vi "Version_4.9_8_on-chip_valves_for25ulSyringe_withModfied_Plunging.vi"() -> ()   [LabVIEW 2020] (continued)
                              tunnel: w4033 -> [w4039]
                              tunnel: w4032 -> [w4038]
                              stop <- w4036 stop-if-true
                              n3656 = Wait (ms)(milliseconds to wait=u32 100) -> ()  [unwired: 1 out]
                              n3657 = stacked-sequence {
                                tunnel: w4041 -> [w4047 _]
                                tunnel: w4040 -> [w4046 w4069]
                                tunnel: w4039 -> [w4045 _]
                                tunnel: w4038 -> [w4044 _]
                                tunnel: [_ w4067] -> w4036
                                frame #0 {
                                n3658 = call "AbsolutePlungerPosition (SubVI).vi"("VISA Refnum in"=w4046) -> ("Plunger Position"=w4043:i32)  [unwired: 10 in]
                                n3659 = case shown="\"Standard Pumping\", Default" w4045 {
                                tunnel: w4047 -> [w4052 w4061]
                                tunnel: w4043 -> [w4053 w4060]
                                tunnel: [w4051 w4058] -> w4042
                                tunnel: w4044 -> [w4050 w4059]
                                frame "Standard Pumping", Default {
                                n3660 = Subtract(x=w4052, y=w4053) -> (x-y=w4049:dbl)
                                n3661 = Absolute Value(x=w4049) -> (abs(x)=w4048:dbl)
                                n3662 = Multiply(x=w4048, y=w4050) -> (x*y=w4055:dbl)
                                n3663 = Divide(x=w4055, y=3000.0) -> (x/y=w4051:dbl)
                                }
                                frame "High Resolution Pumping" {
                                n3664 = Subtract(x=w4061, y=w4060) -> (x-y=w4057:dbl)
                                n3665 = Absolute Value(x=w4057) -> (abs(x)=w4056:dbl)
                                n3666 = Multiply(x=w4056, y=w4059) -> (x*y=w4063:dbl)
                                n3667 = Divide(x=w4063, y=24000.0) -> (x/y=w4058:dbl)
                                }
                                }
                                n3668 = local write "Volume being Injected \nin this process"(w4042) -> ()
                                }
                                frame #1 {
                                n3669 = call "LSPOneStatus (SubVI).vi"("VISA Refnum in"=w4069) -> ("read buffer"=w4071:string)  [unwired: 10 in]
                                n3670 = call <vilib>:"Trim Whitespace.vi"("string"=w4071) -> ("trimmed string"=w4070:string)  [unwired: 1 in]
                                n3671 = Equal?(x=w4070, y="/0`\u0003") -> (x = y?=w4068:bool)
                                n3672 = local read "Stopper that ends \nthe main loops"() -> (w4065:bool)
                                n3673 = local read "Divert Sample \nonto Grid"() -> (w4066:bool)
                                n3674 = Or(x=w4066, y=w4065) -> (x .or. y?=w4064:bool)
                                n3675 = Or(x=w4068, y=w4064) -> (x .or. y?=w4067:bool)
                                }
                              }
                            }
                            n3676 = local read "Stopper that ends \nthe main loops"() -> (w4031:bool)
                            n3677 = case shown="True" w4031 {
                              frame False {
                              }
                              frame True {
                                n3678 = local read "VISA Refnum in\nfor Pump"() -> (w4073:refnum<visa-resource-name>)
                                n3679 = call "HardStopCurrentProcess (SubVI).vi"("VISA Refnum in"=w4073) -> ()  [unwired: 11 in]
                              }
                            }
                          }
                          frame #30 {
                            n3680 = local read "Volume being Injected \nin this process"() -> (w4076:dbl)
                            n3681 = local read "VISA Refnum in\nfor Pump"() -> (w4078:refnum<visa-resource-name>)
                            n3682 = call "AbsolutePlungerPosition (SubVI).vi"("VISA Refnum in"=w4078) -> ("Plunger Position"=w4077:i32)  [unwired: 10 in]
                            n3683 = local write "Pause Data Collection"(TRUE) -> ()
                            n3684 = local write "True Volume being \ninjected in this\nprocess"(w4076) -> ()
                            n3685 = local write "Position\nNow"(w4077) -> ()
                            n3686 = Wait (ms)(milliseconds to wait=u32 500) -> ()  [unwired: 1 out]
                          }
                          frame #31 {
                            # "Sample Deposition onto EM-Grid"
                            n3687 = local read "Divert Sample \nonto Grid"() -> (w4079:bool)
                            n3688 = case shown="True" w4079 {
                              frame False {
                              }
                              frame True {
                                n3689 = stacked-sequence {
                                frame #0 {
                                # "Discard the initial volume of fluid that is present in the channel prior to detection"
                                n3690 = local read "Buffer-C2 Pumping\nResolution"() -> (w4090:T2)
                                n3691 = local read "Initial Plunger Position"() -> (w4089:dbl)
                                n3692 = local read "VISA Refnum in\nfor Pump"() -> (w4091:refnum<visa-resource-name>)
                                n3693 = local read "Position\nNow"() -> (w4087:dbl)
                                n3694 = local read "Volume of Syringe"() -> (w4088:dbl)
                                n3695 = local write "Pause Data Collection"(FALSE) -> ()
                                n3696 = while {
                                tunnel: w4091 -> [w4101]
                                tunnel: w4090 -> [w4100]
                                tunnel: w4089 -> [w4096]
                                tunnel: w4088 -> [w4099]
                                tunnel: w4087 -> [w4095]
                                stop <- w4097 stop-if-true
                                n3697 = stacked-sequence {
                                tunnel: w4101 -> [w4107 w4129 w4159]
                                tunnel: w4100 -> [w4106 w4128 _]
                                tunnel: w4096 -> [w4104 _ _]
                                tunnel: w4099 -> [w4103 w4126 _]
                                tunnel: [_ _ w4152] -> w4097
                                tunnel: w4095 -> [_ w4124 _]
                                frame #0 {
                                # "From here on 'True Volume being injected \nin this process' represents the true total \nvolume in this process"
                                n3698 = call "AbsolutePlungerPosition (SubVI).vi"("VISA Refnum in"=w4107) -> ("Plunger Position"=w4105:i32)  [unwired: 10 in]
                                n3699 = case shown="..\"Standard Pumping\"" w4106 {
                                tunnel: w4105 -> [w4115 w4123]
                                tunnel: w4104 -> [w4114 w4122]
                                tunnel: w4103 -> [w4111 w4119]
                                tunnel: [w4108 w4116] -> w4102
                                frame .."Standard Pumping" {
                                n3700 = Subtract(x=w4115, y=w4114) -> (x-y=w4113:dbl)
                                n3701 = Absolute Value(x=w4113) -> (abs(x)=w4112:dbl)
                                n3702 = Multiply(x=w4112, y=w4111) -> (x*y=w4110:dbl)
                                n3703 = Divide(x=w4110, y=3000.0) -> (x/y=w4108:dbl)
                                }
                                frame "High Resolution Pumping".. {
                                n3704 = Subtract(x=w4123, y=w4122) -> (x-y=w4121:dbl)
                                n3705 = Absolute Value(x=w4121) -> (abs(x)=w4120:dbl)
                                n3706 = Multiply(x=w4120, y=w4119) -> (x*y=w4118:dbl)
                                n3707 = Divide(x=w4118, y=24000.0) -> (x/y=w4116:dbl)
                                }
                                }
                                n3708 = local write "True Volume being \ninjected in this\nprocess"(w4102) -> ()
                                }
                                frame #1 {
                                # "From here on 'Volume being injected \nin this process' represents the volume \nin this sub process"
                                n3709 = call "AbsolutePlungerPosition (SubVI).vi"("VISA Refnum in"=w4129) -> ("Plunger Position"=w4127:i32)  [unwired: 10 in]
                                n3710 = case shown="..\"Standard Pumping\"" w4128 {
                                tunnel: w4127 -> [w4137 w4145]
                                tunnel: w4124 -> [w4136 w4144]
                                tunnel: w4126 -> [w4133 w4141]
                                tunnel: [w4130 w4138] -> w4125
                                frame .."Standard Pumping" {
                                n3711 = Subtract(x=w4137, y=w4136) -> (x-y=w4135:dbl)
                                n3712 = Absolute Value(x=w4135) -> (abs(x)=w4134:dbl)
                                n3713 = Multiply(x=w4134, y=w4133) -> (x*y=w4132:dbl)
                                n3714 = Divide(x=w4132, y=3000.0) -> (x/y=w4130:dbl)
                                }
                                frame "High Resolution Pumping".. {
                                n3715 = Subtract(x=w4145, y=w4144) -> (x-y=w4143:dbl)
                                n3716 = Absolute Value(x=w4143) -> (abs(x)=w4142:dbl)
                                n3717 = Multiply(x=w4142, y=w4141) -> (x*y=w4140:dbl)
                                n3718 = Divide(x=w4140, y=24000.0) -> (x/y=w4138:dbl)
                                }
                                }
                                n3719 = local write "Volume being Injected \nin this process"(w4125) -> ()
                                }
                                frame #2 {
                                n3720 = local read "Discard Volume"() -> (w4146:dbl)
                                n3721 = local read "Discard fluid \nprior to 1st \ndeposition"() -> (w4151:bool)
                                n3722 = local read "Volume being Injected \nin this process"() -> (w4150:dbl)
                                n3723 = Greater Or Equal?(x=w4150, y=w4146) -> (x >= y?=w4148:bool)
                                n3724 = call "AbsolutePlungerPositionStatus (SubVI).vi"("VISA Refnum in"=w4159) -> ("read buffer"=w4158:string)  [unwired: 10 in]
                                n3725 = local read "Stop for End of \nExperiment \nand Data Writing"() -> (w4155:bool)
                                n3726 = call <vilib>:"Trim Whitespace.vi"("string"=w4158) -> ("trimmed string"=w4157:string)  [unwired: 1 in]
                                n3727 = Not(x=w4151) -> (.not. x?=w4149:bool)
                                n3728 = Equal?(x=w4157, y="/0`\u0003") -> (x = y?=w4154:bool)
                                n3729 = Or(x=w4149, y=w4148) -> (x .or. y?=w4147:bool)
                                n3730 = Or(x=w4147, y=w4155) -> (x .or. y?=w4153:bool)
                                n3731 = Or(x=w4154, y=w4153) -> (x .or. y?=w4152:bool)
                                }
                                }
                                n3732 = Wait (ms)(milliseconds to wait=u32 100) -> ()  [unwired: 1 out]
                                }
                                n3733 = local write "Valve V4 Open"(TRUE ("Valve V4 Open")) -> ()
                                n3734 = local write "Valve V3 Open"(FALSE ("Valve V3 Open")) -> ()
                                n3735 = local write "Valve V2 Open"(FALSE ("Valve V2 Open")) -> ()
                                n3736 = local write "Valve V1 Open"(FALSE ("Valve V1 Open")) -> ()
                                n3737 = local write "Valve V5 Open"(TRUE ("Valve V5 Open")) -> ()
                                n3738 = local write "Valve V6 Open"(TRUE ("Valve V6 Open")) -> ()
                                n3739 = local write "Valve V7 Open"(FALSE ("Valve V7 Open")) -> ()
                                n3740 = local write "Volume being Injected \nin this process"(0.0) -> ()
                                }
                                frame #1 {
                                # "Keeps the on-chip valve V1, V2 and V3 closed,\nHalts also deposition onto the grid\nand waits for the 1st redeposit command. Once the command is issued\nit starts pumpoing and moves onto the next frame"
                                n3741 = stacked-sequence {
                                frame #0 {
                                n3742 = local write "Valve V5 Open"(FALSE ("Valve V5 Open")) -> ()
                                n3743 = local write "Valve V1 Open"(FALSE ("Valve V1 Open")) -> ()
                                n3744 = local read "VISA Refnum in\nfor Pump"() -> (w4169:refnum<visa-resource-name>)
                                n3745 = local write "Valve V2 Open"(FALSE ("Valve V2 Open")) -> ()
                                n3746 = local write "Valve V6 Open"(FALSE ("Valve V6 Open")) -> ()
                                n3747 = local write "Re-deposit Sample\nonto Grid"(FALSE ("Redeposit Sample\nonto Grid")) -> ()
                                n3748 = local write "Pause Data Collection"(TRUE ("Pause Data Collection")) -> ()
                                n3749 = call "HardStopCurrentProcess (SubVI).vi"("VISA Refnum in"=w4169) -> ()  [unwired: 11 in]
                                n3750 = local write "Valve V7 Open"(FALSE ("Valve V7 Open")) -> ()
                                n3751 = local write "Valve V3 Open"(FALSE ("Valve V3 Open")) -> ()
                                n3752 = local write "Valve V4 Open"(FALSE ("Valve V4 Open")) -> ()
                                }
                                frame #1 {
                                n3753 = while {
                                stop <- w4172 stop-if-true
                                n3754 = local read "Stop for End of \nExperiment \nand Data Writing"() -> (w4173:bool)
                                n3755 = local read "Re-deposit Sample\nonto Grid"() -> (w4174:bool)
                                n3756 = Or(x=w4174, y=w4173) -> (x .or. y?=w4172:bool)
                                }
                                n3757 = local write "Discard fluid \nprior to 1st \ndeposition"(FALSE ("Discard fluid \nprior to 1st \ndeposition")) -> ()
                                n3758 = One Button Dialog(message="Do you want to deposit sample on another grid? If yes, turn on 'Re-deposit Sample onto Grid'. Else turn on STOP ") -> ()  [unwired: 1 in, 1 out]
                                }
                                frame #2 {
                                n3759 = local write "Valve V6 Open"(TRUE ("Valve V3 Open")) -> ()
                                n3760 = local write "Valve V4 Open"(TRUE ("Valve V1 Open")) -> ()
                                n3761 = local write "Valve V5 Open"(TRUE ("Valve V2 Open")) -> ()
                                n3762 = local write "Valve V7 Open"(FALSE ("Valve V7 Open")) -> ()
                                }
                                frame #3 {
                                n3763 = local read "Re-deposit Sample\nonto Grid"() -> (w4179:bool)
                                n3764 = case shown="True" w4179 {
                                frame False {
                                n3765 = local write "Suction On/Off"(FALSE ("Suction On/Off")) -> ()
                                }
                                frame True {
                                n3766 = stacked-sequence {
                                frame #0 {
                                n3767 = local read "VISA Refnum in\nfor Pump"() -> (w4182:refnum<visa-resource-name>)
                                n3768 = call "AbsolutePlungerPosition (SubVI).vi"("VISA Refnum in"=w4182) -> ("Plunger Position"=w4181:i32)  [unwired: 10 in]
                                n3769 = local write "Position\nNow"(w4181) -> ()
                                }
                                frame #1 {
                                n3770 = local read "Buffer-C2 Pumping\nResolution"() -> (w4184:T2)
                                n3771 = case shown="\"Standard Pumping\", Default" w4184 {
                                tunnel: [w4185 w4196] -> w4183
                                frame "Standard Pumping", Default {
                                n3772 = local read "Buffer-C2 Volume \nto be Pumped"() -> (w4188:dbl)
                                n3773 = local read "Volume of Syringe"() -> (w4191:dbl)
                                n3774 = local read "Initial Plunger Position"() -> (w4195:dbl)
                                n3775 = local read "Position\nNow"() -> (w4194:dbl)
                                n3776 = Subtract(x=w4195, y=w4194) -> (x-y=w4193:dbl)
                                n3777 = Absolute Value(x=w4193) -> (abs(x)=w4192:dbl)
                                n3778 = Multiply(x=w4192, y=w4191) -> (x*y=w4190:dbl)
                                n3779 = Divide(x=w4190, y=3000.0) -> (x/y=w4187:dbl)
                                n3780 = Subtract(x=w4187, y=w4188) -> (x-y=w4186:dbl)
                                n3781 = Absolute Value(x=w4186) -> (abs(x)=w4185:dbl)
                                }
                                frame "High Resolution Pumping" {
                                n3782 = local read "Buffer-C2 Volume \nto be Pumped"() -> (w4199:dbl)
                                n3783 = local read "Volume of Syringe"() -> (w4202:dbl)
                                n3784 = local read "Initial Plunger Position"() -> (w4206:dbl)
                                n3785 = local read "Position\nNow"() -> (w4205:dbl)
                                n3786 = Subtract(x=w4206, y=w4205) -> (x-y=w4204:dbl)
                                n3787 = Absolute Value(x=w4204) -> (abs(x)=w4203:dbl)
                                n3788 = Multiply(x=w4203, y=w4202) -> (x*y=w4201:dbl)
                                n3789 = Divide(x=w4201, y=24000.0) -> (x/y=w4198:dbl)
                                n3790 = Subtract(x=w4198, y=w4199) -> (x-y=w4197:dbl)
                                n3791 = Absolute Value(x=w4197) -> (abs(x)=w4196:dbl)
                                }
                                }
                                n3792 = local write "Buffer-C Volume\nleft to be Pumped"(w4183) -> ()
                                }
                                frame #2 {
                                n3793 = local read "Buffer-C2 Dispense\nFlow Rate (ul/min)"() -> (w4210:dbl)
                                n3794 = local read "Buffer-C2 Pumping\nResolution"() -> (w4209:T2)
                                n3795 = local read "VISA Refnum in\nfor Pump"() -> (w4212:refnum<visa-resource-name>)
                                n3796 = local read "Volume of Syringe"() -> (w4211:dbl)
                                n3797 = call "GoToAbsolutePosition(SubVI).vi"("Absolute Volume Position in Syringe (in ul)"=0.0, "Volume of Syringe"=w4211, "Resolution of Pumping"=w4209, "Flow Rate (ul/min)"=w4210, "VISA Refnum in"=w4212) -> ()  [unwired: 6 in, 1 out]
                                n3798 = local write "Suction On/Off"(FALSE ("Suction On/Off")) -> ()
                                }
                                }
                                }
                                }
                                }
                                frame #4 {
                                n3799 = local read "Stop for End of \nExperiment \nand Data Writing"() -> (w4213:bool)
                                n3800 = case shown="True" w4213 {
                                frame False {
                                }
                                frame True {
                                n3801 = local read "VISA Refnum in\nfor Pump"() -> (w4214:refnum<visa-resource-name>)
                                n3802 = call "HardStopCurrentProcess (SubVI).vi"("VISA Refnum in"=w4214) -> ()  [unwired: 11 in]
                                }
                                }
                                }
                                }
                                }
                                frame #2 {
                                # "Keeps the on-chip valve V1, V2 Open and V3 closed"
                                n3803 = while {
                                stop <- w4218 stop-if-true
                                n3804 = local read "Suction On/Off"() -> (w4219:bool)
                                n3805 = case shown="True" w4219 {
                                frame False {
                                n3806 = local read "Buffer-C2 Pumping\nResolution"() -> (w4225:T2)
                                n3807 = local read "Initial Plunger Position"() -> (w4224:dbl)
                                n3808 = local read "VISA Refnum in\nfor Pump"() -> (w4226:refnum<visa-resource-name>)
                                n3809 = local read "Position\nNow"() -> (w4222:dbl)
                                n3810 = local read "Volume of Syringe"() -> (w4223:dbl)
                                n3811 = local write "Volume being Injected \nin this process"(0.0) -> ()
                                n3812 = local write "Pause Data Collection"(FALSE) -> ()
                                n3813 = while {
                                tunnel: w4226 -> [w4233]
                                tunnel: w4225 -> [w4232]
                                tunnel: w4224 -> [w4228]
                                tunnel: w4223 -> [w4231]
                                tunnel: w4222 -> [w4227]
                                stop <- w4229 stop-if-true
                                n3814 = stacked-sequence {
                                tunnel: w4233 -> [w4239 w4261 w4286]
                                tunnel: w4232 -> [w4238 w4260 _]
                                tunnel: w4228 -> [w4236 _ _]
                                tunnel: w4231 -> [w4235 w4258 _]
                                tunnel: [_ _ w4278] -> w4229
                                tunnel: w4227 -> [_ w4256 _]
                                frame #0 {
                                # "From here on 'True Volume being injected \nin this process' represents the true total \nvolume in this process"
                                n3815 = call "AbsolutePlungerPosition (SubVI).vi"("VISA Refnum in"=w4239) -> ("Plunger Position"=w4237:i32)  [unwired: 10 in]
                                n3816 = case shown="..\"Standard Pumping\"" w4238 {
                                tunnel: w4237 -> [w4247 w4255]
                                tunnel: w4236 -> [w4246 w4254]
                                tunnel: w4235 -> [w4243 w4251]
                                tunnel: [w4240 w4248] -> w4234
                                frame .."Standard Pumping" {
                                n3817 = Subtract(x=w4247, y=w4246) -> (x-y=w4245:dbl)
                                n3818 = Absolute Value(x=w4245) -> (abs(x)=w4244:dbl)
                                n3819 = Multiply(x=w4244, y=w4243) -> (x*y=w4242:dbl)
                                n3820 = Divide(x=w4242, y=3000.0) -> (x/y=w4240:dbl)
                                }
                                frame "High Resolution Pumping".. {
                                n3821 = Subtract(x=w4255, y=w4254) -> (x-y=w4253:dbl)
                                n3822 = Absolute Value(x=w4253) -> (abs(x)=w4252:dbl)
                                n3823 = Multiply(x=w4252, y=w4251) -> (x*y=w4250:dbl)
                                n3824 = Divide(x=w4250, y=24000.0) -> (x/y=w4248:dbl)
                                }
                                }
                                n3825 = local write "True Volume being \ninjected in this\nprocess"(w4234) -> ()
                                }
                                frame #1 {
                                # "From here on 'Volume being injected \nin this process' represents the volume \nin this sub process"
                                n3826 = call "AbsolutePlungerPosition (SubVI).vi"("VISA Refnum in"=w4261) -> ("Plunger Position"=w4259:i32)  [unwired: 10 in]
                                n3827 = case shown="..\"Standard Pumping\"" w4260 {
                                tunnel: w4259 -> [w4269 w4277]
                                tunnel: w4256 -> [w4268 w4276]
                                tunnel: w4258 -> [w4265 w4273]
                                tunnel: [w4262 w4270] -> w4257
                                frame .."Standard Pumping" {
                                n3828 = Subtract(x=w4269, y=w4268) -> (x-y=w4267:dbl)
                                n3829 = Absolute Value(x=w4267) -> (abs(x)=w4266:dbl)
                                n3830 = Multiply(x=w4266, y=w4265) -> (x*y=w4264:dbl)
                                n3831 = Divide(x=w4264, y=3000.0) -> (x/y=w4262:dbl)
                                }
                                frame "High Resolution Pumping".. {
                                n3832 = Subtract(x=w4277, y=w4276) -> (x-y=w4275:dbl)
                                n3833 = Absolute Value(x=w4275) -> (abs(x)=w4274:dbl)
                                n3834 = Multiply(x=w4274, y=w4273) -> (x*y=w4272:dbl)
                                n3835 = Divide(x=w4272, y=24000.0) -> (x/y=w4270:dbl)
                                }
                                }
                                n3836 = local write "Volume being Injected \nin this process"(w4257) -> ()
                                }
                                frame #2 {
                                n3837 = local read "Stop for End of \nExperiment \nand Data Writing"() -> (w4281:bool)
                                n3838 = local read "Suction On/Off"() -> (w4282:bool)
                                n3839 = call "AbsolutePlungerPositionStatus (SubVI).vi"("VISA Refnum in"=w4286) -> ("read buffer"=w4285:string)  [unwired: 10 in]
                                n3840 = call <vilib>:"Trim Whitespace.vi"("string"=w4285) -> ("trimmed string"=w4284:string)  [unwired: 1 in]
                                n3841 = Equal?(x=w4284, y="/0`\u0003") -> (x = y?=w4280:bool)
                                n3842 = Or(x=w4282, y=w4281) -> (x .or. y?=w4279:bool)
                                n3843 = Or(x=w4280, y=w4279) -> (x .or. y?=w4278:bool)
                                }
                                }
                                n3844 = Wait (ms)(milliseconds to wait=u32 100) -> ()  [unwired: 1 out]
                                }
                                }
                                frame True {
                                n3845 = stacked-sequence {
                                frame #0 {
                                n3846 = local read "Suction Pressure\nfor EM-grid \nDeposition (mbar)"() -> (w4291:sgl)
                                n3847 = local write "Valve V4 Open"(FALSE ("Valve V4 Open")) -> ()
                                n3848 = local read "VISA Refnum in\nfor Pump"() -> (w4294:refnum<visa-resource-name>)
                                n3849 = local write "Valve V5 Open"(FALSE ("Valve V1 Open")) -> ()
                                n3850 = local write "Suction pressure \nfor grid deposition"(w4291) -> ()
                                n3851 = local write "Re-deposit Sample\nonto Grid"(FALSE ("Redeposit Sample\nonto Grid")) -> ()
                                n3852 = local write "Pause Data Collection"(TRUE ("Pause Data Collection")) -> ()
                                n3853 = call "HardStopCurrentProcess (SubVI).vi"("VISA Refnum in"=w4294) -> ()  [unwired: 11 in]
                                n3854 = local write "Valve V6 Open"(TRUE ("Valve V2 Open")) -> ()
                                n3855 = local write "Valve V7 Open"(TRUE ("Valve V3 Open")) -> ()
                                }
                                frame #1 {
                                n3856 = call <vilib>:"fgt init.vi"() -> ("error out"=w4295:errorcluster)  [unwired: 11 in]
                                n3857 = while {
                                tunnel: [w4299] -> w4296
                                tunnel: w4295 -> [w4298]
                                stop <- w4302 stop-if-true
                                # "'5' corresponds to 2nd positin in the line-up series"
                                n3858 = local read "Suction On/Off"() -> (w4297:bool)
                                n3859 = local read "Stop for End of \nExperiment \nand Data Writing"() -> (w4303:bool)
                                n3860 = case shown="True" w4297 {
                                tunnel: [0 w4308] -> w4300
                                frame False {
                                }
                                frame True {
                                n3861 = local read "Suction Pressure\nfor EM-grid \nDeposition (mbar)"() -> (w4308:sgl)
                                }
                                }
                                n3862 = call <vilib>:"fgt set pressure.vi"("error in (no error)"=w4298, "pressure"=w4300, "pressureIndex"=u32 1) -> ("error out"=w4299:errorcluster)  [unwired: 8 in]
                                n3863 = local read "Suction On/Off"() -> (w4305:bool)
                                n3864 = Not(x=w4305) -> (.not. x?=w4304:bool)
                                n3865 = Wait (ms)(milliseconds to wait=u32 100) -> ()  [unwired: 1 out]
                                n3866 = Or(x=w4304, y=w4303) -> (x .or. y?=w4302:bool)
                                }
                                n3867 = call <vilib>:"fgt close.vi"("error in (no error)"=w4296) -> ()  [unwired: 10 in, 1 out]
                                }
                                frame #2 {
                                n3868 = local write "Valve V7 Open"(FALSE ("Valve V3 Open")) -> ()
                                n3869 = local write "Valve V5 Open"(FALSE ("Valve V1 Open")) -> ()
                                n3870 = local write "Valve V6 Open"(FALSE ("Valve V2 Open")) -> ()
                                n3871 = local write "Valve V4 Open"(FALSE ("Valve V4 Open")) -> ()
                                }
                                frame #3 {
                                n3872 = while {
                                stop <- w4314 stop-if-true
                                n3873 = local read "Stop for End of \nExperiment \nand Data Writing"() -> (w4315:bool)
                                n3874 = local read "Re-deposit Sample\nonto Grid"() -> (w4316:bool)
                                n3875 = Or(x=w4316, y=w4315) -> (x .or. y?=w4314:bool)
                                }
                                n3876 = One Button Dialog(message="Do you want to deposit sample on another grid? If yes, turn on 'Re-deposit Sample onto Grid'. Else turn on STOP ") -> ()  [unwired: 1 in, 1 out]
                                }
                                frame #4 {
                                n3877 = local write "Valve V4 Open"(TRUE ("Valve V4 Open")) -> ()
                                n3878 = local write "Valve V7 Open"(FALSE ("Valve V3 Open")) -> ()
                                n3879 = local write "Valve V5 Open"(TRUE ("Valve V1 Open")) -> ()
                                n3880 = local write "Valve V6 Open"(TRUE ("Valve V2 Open")) -> ()
                                }
                                frame #5 {
                                n3881 = local read "Re-deposit Sample\nonto Grid"() -> (w4321:bool)
                                n3882 = case shown="False" w4321 {
                                frame False {
                                n3883 = local write "Suction On/Off"(FALSE ("Suction On/Off")) -> ()
                                }
                                frame True {
                                n3884 = stacked-sequence {
                                frame #0 {
                                n3885 = local read "VISA Refnum in\nfor Pump"() -> (w4324:refnum<visa-resource-name>)
                                n3886 = call "AbsolutePlungerPosition (SubVI).vi"("VISA Refnum in"=w4324) -> ("Plunger Position"=w4323:i32)  [unwired: 10 in]
                                n3887 = local write "Position\nNow"(w4323) -> ()
                                }
                                frame #1 {
                                n3888 = local read "Buffer-C2 Pumping\nResolution"() -> (w4326:T2)
                                n3889 = case shown="\"Standard Pumping\", Default" w4326 {
                                tunnel: [w4327 w4338] -> w4325
                                frame "Standard Pumping", Default {
                                n3890 = local read "Buffer-C2 Volume \nto be Pumped"() -> (w4330:dbl)
                                n3891 = local read "Volume of Syringe"() -> (w4333:dbl)
                                n3892 = local read "Initial Plunger Position"() -> (w4337:dbl)
                                n3893 = local read "Position\nNow"() -> (w4336:dbl)
                                n3894 = Subtract(x=w4337, y=w4336) -> (x-y=w4335:dbl)
                                n3895 = Absolute Value(x=w4335) -> (abs(x)=w4334:dbl)
                                n3896 = Multiply(x=w4334, y=w4333) -> (x*y=w4332:dbl)
                                n3897 = Divide(x=w4332, y=3000.0) -> (x/y=w4329:dbl)
                                n3898 = Subtract(x=w4329, y=w4330) -> (x-y=w4328:dbl)
                                n3899 = Absolute Value(x=w4328) -> (abs(x)=w4327:dbl)
                                }
                                frame "High Resolution Pumping" {
                                n3900 = local read "Buffer-C2 Volume \nto be Pumped"() -> (w4341:dbl)
                                n3901 = local read "Volume of Syringe"() -> (w4344:dbl)
                                n3902 = local read "Initial Plunger Position"() -> (w4348:dbl)
                                n3903 = local read "Position\nNow"() -> (w4347:dbl)
                                n3904 = Subtract(x=w4348, y=w4347) -> (x-y=w4346:dbl)
                                n3905 = Absolute Value(x=w4346) -> (abs(x)=w4345:dbl)
                                n3906 = Multiply(x=w4345, y=w4344) -> (x*y=w4343:dbl)
                                n3907 = Divide(x=w4343, y=24000.0) -> (x/y=w4340:dbl)
                                n3908 = Subtract(x=w4340, y=w4341) -> (x-y=w4339:dbl)
                                n3909 = Absolute Value(x=w4339) -> (abs(x)=w4338:dbl)
                                }
                                }
                                n3910 = local write "Buffer-C Volume\nleft to be Pumped"(w4325) -> ()
                                }
                                frame #2 {
                                n3911 = local read "Buffer-C2 Dispense\nFlow Rate (ul/min)"() -> (w4352:dbl)
                                n3912 = local read "Buffer-C2 Pumping\nResolution"() -> (w4351:T2)
                                n3913 = local read "VISA Refnum in\nfor Pump"() -> (w4354:refnum<visa-resource-name>)
                                n3914 = local read "Volume of Syringe"() -> (w4353:dbl)
                                n3915 = call "GoToAbsolutePosition(SubVI).vi"("Absolute Volume Position in Syringe (in ul)"=0.0, "Volume of Syringe"=w4353, "Resolution of Pumping"=w4351, "Flow Rate (ul/min)"=w4352, "VISA Refnum in"=w4354) -> ()  [unwired: 6 in, 1 out]
                                n3916 = local write "Suction On/Off"(FALSE ("Suction On/Off")) -> ()
                                }
                                }
                                }
                                }
                                }
                                frame #6 {
                                n3917 = local read "Stop for End of \nExperiment \nand Data Writing"() -> (w4355:bool)
                                n3918 = case shown="True" w4355 {
                                frame False {
                                }
                                frame True {
                                n3919 = local read "VISA Refnum in\nfor Pump"() -> (w4356:refnum<visa-resource-name>)
                                n3920 = call "HardStopCurrentProcess (SubVI).vi"("VISA Refnum in"=w4356) -> ()  [unwired: 11 in]
                                }
                                }
                                }
                                }
                                }
                                }
                                n3921 = local read "Stop for End of \nExperiment \nand Data Writing"() -> (w4217:bool)
                                n3922 = local read "Divert Sample \nonto Grid"() -> (w4216:bool)
                                n3923 = Not(x=w4216) -> (.not. x?=w4215:bool)
                                n3924 = Or(x=w4215, y=w4217) -> (x .or. y?=w4218:bool)
                                }
                                }
                                }
                                n3925 = local write "Discard fluid \nprior to 1st \ndeposition"(TRUE ("Discard fluid \nprior to 1st \ndeposition")) -> ()
                              }
                            }
                          }
                          frame #32 {
                            n3926 = local write "Valve V2 Open"(FALSE ("Valve V2 Open")) -> ()
                            n3927 = local write "Valve V4 Open"(FALSE ("Valve V4 Open")) -> ()
                            n3928 = local write "Valve V3 Open"(FALSE ("Valve V3 Open")) -> ()
                            n3929 = local write "Valve V1 Open"(FALSE ("Valve V1 Open")) -> ()
                            n3930 = local write "Valve V6 Open"(FALSE ("Valve V6 Open")) -> ()
                            n3931 = local write "Valve V5 Open"(FALSE ("Valve V5 Open")) -> ()
                            n3932 = local write "Valve V7 Open"(FALSE ("Valve V7 Open")) -> ()
                            n3933 = local read "VISA Refnum in\nfor Valve"() -> (w4361:refnum<visa-resource-name>)
                            n3934 = local read "External Valve \nOPEN"() -> (w4360:string)
                            n3935 = Wait (ms)(milliseconds to wait=u32 500) -> ()  [unwired: 1 out]
                            n3936 = call "PortChanger_Valve (SubVI).vi"("Port Number"=w4360, "VISA Refnum in"=w4361) -> ()  [unwired: 10 in]
                          }
                          frame #33 {
                            n3937 = local read "Stopper that ends \nthe main loops"() -> (w4368:bool)
                            n3938 = Wait (ms)(milliseconds to wait=u32 500) -> ()  [unwired: 1 out]
                            n3939 = case shown="True" w4368 {
                              frame False {
                              }
                              frame True {
                                n3940 = local read "VISA Refnum in\nfor Pump"() -> (w4372:refnum<visa-resource-name>)
                                n3941 = call "HardStopCurrentProcess (SubVI).vi"("VISA Refnum in"=w4372) -> ()  [unwired: 11 in]
                              }
                            }
                            n3942 = local write "Pause Data Collection"(TRUE ("Pause Data Collection")) -> ()
                            n3943 = local write "Start the Process"(FALSE ("Start the Process")) -> ()
                            n3944 = local write "Divert Sample \nonto Grid"(FALSE ("Divert Sample \nonto Grid")) -> ()
                          }
                          frame #34 {
                            n3945 = local write "Volume being Injected \nin this process"(0.0 ("Volume being Injected \nin this process")) -> ()
                            n3946 = local write "Elution of Column-2"(FALSE ("Elution of Column-2")) -> ()
                            n3947 = local write "SEC On"(FALSE ("SEC On")) -> ()
                          }
                        }
                      }
                    }
                  }
                }
              }
              frame True {
                n3948 = local write "Pause Data Collection"(FALSE ("Pause Data Collection")) -> ()
              }
            }
          }
          frame "Automated Protein Purification with Re-SEC Possibility, 8 SOD Valves and On/Off External Valve" {
            n3949 = local read "Stopper that ends \nthe main loops"() -> (w4377:bool)
            n3950 = case shown="False" w4377 {
              frame False {
                n3951 = local read "Start the Process"() -> (w4378:bool)
                n3952 = case shown="True" w4378 {
                  frame False {
                    n3953 = local read "Stopper that ends \nthe main loops"() -> (w4380:bool)
                    n3954 = local read "Start the Process"() -> (w4379:bool)
                    n3955 = Or(x=w4380, y=w4379) -> (x .or. y?=w4381:bool)
                    n3956 = case shown="False" w4381 {
                      frame False {
                        n3957 = while {
                          stop <- w4384 stop-if-true
                          n3958 = local read "Stop for End of \nExperiment \nand Data Writing"() -> (w4383:bool)
                          n3959 = local read "Stopper that ends \nthe main loops"() -> (w4386:bool)
                          n3960 = local read "Start the Process"() -> (w4385:bool)
                          n3961 = Wait (ms)(milliseconds to wait=u32 10) -> ()  [unwired: 1 out]
                          n3962 = Or(x=w4386, y=w4385) -> (x .or. y?=w4384:bool)
                          n3963 = local write "Stopper that ends \nthe main loops"(w4383) -> ()
                        }
                        n3964 = One Button Dialog(message="Please Select the Process and Press 'Start the Process' Button") -> ()  [unwired: 1 in, 1 out]
                      }
                      frame True {
                      }
                    }
                  }
                  frame True {
                    n3965 = stacked-sequence {
                      frame #0 {
                        # "Equilibrate Column-1 with Buffer-A obtained from port-4 and pumped via port-2 and Column-2 with Buffer-C obtained from port-4 and pumped onto chip via port-6 onto the chip ...with an initial and inbetween wash of tubings while changing the buffers"
                        n3966 = stacked-sequence {
                          frame #0 {
                            n3967 = local write "Equilibriating \nColumn-1"(TRUE ("Equilibriating \nColumn-1")) -> ()
                            n3968 = local write "External Valve \nOpen"(FALSE ("External Valve \nOpen")) -> ()
                            n3969 = local write "Valve V4 Open"(FALSE ("Valve V4 Open")) -> ()
                            n3970 = local write "Valve V1 Open"(FALSE ("Valve V1 Open")) -> ()
                            n3971 = local write "Valve V2 Open"(FALSE ("Valve V2 Open")) -> ()
                            n3972 = local write "Valve V3 Open"(FALSE ("Valve V3 Open")) -> ()
                            n3973 = local write "Valve V7 Open"(FALSE ("Valve V7 Open")) -> ()
                            n3974 = local write "Valve V8 Open"(FALSE ("Valve V8 Open")) -> ()
                            n3975 = local write "Valve V5 Open"(FALSE ("Valve V5 Open")) -> ()
                            n3976 = local write "Valve V6 Open"(FALSE ("Valve V6 Open")) -> ()
                            n3977 = call <vilib>:"fgt init.vi"() -> ("error out"=w4392:errorcluster)  [unwired: 11 in]
                            n3978 = while {
                              tunnel: w4392 -> [w4401]
                              tunnel: [w4400] -> w4391
                              stop <- w4404 stop-if-true
                              # "Keeping the valve closing pressure of push pull to zero"
                              n3979 = local read "Stop for End of \nExperiment \nand Data Writing"() -> (w4405:bool)
                              n3980 = local read "Equilibriating \nColumn-1"() -> (w4406:bool)
                              n3981 = call <vilib>:"fgt set pressure.vi"("error in (no error)"=w4401, "pressure"=sgl 0.0 ("order"), "pressureIndex"=1 ("module")) -> ("error out"=w4400:errorcluster)  [unwired: 8 in]
                              n3982 = Or(x=w4406, y=w4405) -> (x .or. y?=w4404:bool)
                              n3983 = Wait (ms)(milliseconds to wait=u32 10) -> ()  [unwired: 1 out]
                            }
                            n3984 = call <vilib>:"fgt close.vi"("error in (no error)"=w4391) -> ()  [unwired: 10 in, 1 out]
                          }
                          frame #1 {
                            # "Clean the elution tubing with Buffer-B1"
                            n3985 = local read "N-B1"() -> (w4408:i32)
                            n3986 = for {
                              N: w4408 -> [_]
                              n3987 = stacked-sequence {
                                frame #0 {
                                n3988 = local read "VISA Refnum in\nfor Pump"() -> (w4411:refnum<visa-resource-name>)
                                n3989 = local read "Port for \nB-Elution"() -> (w4410:string)
                                n3990 = call "PortChanger (SubVI).vi"("Port Number"=w4410, "VISA Refnum in"=w4411) -> ()  [unwired: 10 in]
                                }
                                frame #1 {
                                n3991 = local read "VISA Refnum in\nfor Pump"() -> (w4412:refnum<visa-resource-name>)
                                n3992 = call "ProcessCompletionWaiter (SubVI).vi"("VISA Refnum in"=w4412) -> ()  [unwired: 11 in]
                                }
                                frame #2 {
                                n3993 = local read "VISA Refnum in\nfor Pump"() -> (w4417:refnum<visa-resource-name>)
                                n3994 = local read "Apparent Volume\nof Syringe"() -> (w4413:dbl)
                                n3995 = local read "Volume of Syringe"() -> (w4414:dbl)
                                n3996 = call "RPickUp(SubVI).vi"("Volume to be picked up"=w4413, "Volume of Syringe"=w4414, "Resolution of PickUP"=T2."Standard Pumping", "PickUp Flow Rate (ul/min)"=150.0, "VISA Refnum in"=w4417) -> ()  [unwired: 6 in, 1 out]
                                }
                                frame #3 {
                                n3997 = local read "Stopper that ends \nthe main loops"() -> (w4418:bool)
                                n3998 = local read "VISA Refnum in\nfor Pump"() -> (w4419:refnum<visa-resource-name>)
                                n3999 = case shown="True" w4418 {
                                frame False {
                                }
                                frame True {
                                n4000 = local read "VISA Refnum in\nfor Pump"() -> (w4420:refnum<visa-resource-name>)
                                n4001 = call "HardStopCurrentProcess (SubVI).vi"("VISA Refnum in"=w4420) -> ()  [unwired: 11 in]
                                }
                                }
                                n4002 = call "ProcessCompletionWaiter (SubVI).vi"("VISA Refnum in"=w4419) -> ()  [unwired: 11 in]
                                }
                                frame #4 {
                                n4003 = local read "VISA Refnum in\nfor Pump"() -> (w4422:refnum<visa-resource-name>)
                                n4004 = call "PortChanger (SubVI).vi"("Port Number"="1", "VISA Refnum in"=w4422) -> ()  [unwired: 10 in]
                                }
                                frame #5 {
                                n4005 = local read "Stopper that ends \nthe main loops"() -> (w4423:bool)
                                n4006 = local read "VISA Refnum in\nfor Pump"() -> (w4424:refnum<visa-resource-name>)
                                n4007 = case shown="True" w4423 {
                                frame False {
                                }
                                frame True {
                                n4008 = local read "VISA Refnum in\nfor Pump"() -> (w4425:refnum<visa-resource-name>)
                                n4009 = call "HardStopCurrentProcess (SubVI).vi"("VISA Refnum in"=w4425) -> ()  [unwired: 11 in]
                                }
                                }
                                n4010 = call "ProcessCompletionWaiter (SubVI).vi"("VISA Refnum in"=w4424) -> ()  [unwired: 11 in]
                                }
                                frame #6 {
                                n4011 = local read "VISA Refnum in\nfor Pump"() -> (w4430:refnum<visa-resource-name>)
                                n4012 = local read "Volume of Syringe"() -> (w4427:dbl)
                                n4013 = call "GoToAbsolutePosition(SubVI).vi"("Absolute Volume Position in Syringe (in ul)"=0.0 ("Volume to be picked up"), "Volume of Syringe"=w4427, "Resolution of Pumping"=T2."Standard Pumping" ("Resolution of PickUP"), "Flow Rate (ul/min)"=150.0 ("PickUp Flow Rate (ul/min)"), "VISA Refnum in"=w4430) -> ()  [unwired: 6 in, 1 out]
                                }
                                frame #7 {
                                n4014 = local read "Stopper that ends \nthe main loops"() -> (w4431:bool)
                                n4015 = local read "VISA Refnum in\nfor Pump"() -> (w4432:refnum<visa-resource-name>)
                                n4016 = case shown="True" w4431 {
                                frame False {
                                }
                                frame True {
                                n4017 = local read "VISA Refnum in\nfor Pump"() -> (w4433:refnum<visa-resource-name>)
                                n4018 = call "HardStopCurrentProcess (SubVI).vi"("VISA Refnum in"=w4433) -> ()  [unwired: 11 in]
                                }
                                }
                                n4019 = call "ProcessCompletionWaiter (SubVI).vi"("VISA Refnum in"=w4432) -> ()  [unwired: 11 in]
                                }
                              }
                              n4020 = local write "Pause Data Collection"(TRUE ("Pause Data Collection")) -> ()
                            }
                          }
                          frame #2 {
                            # "Switch to Port-7"
                            # "Port-7 of pump is connected to Buffer-B"
                            n4021 = local read "VISA Refnum in\nfor Pump"() -> (w4435:refnum<visa-resource-name>)
                            n4022 = local read "Port for \nB-Elution"() -> (w4434:string)
                            n4023 = call "PortChanger (SubVI).vi"("Port Number"=w4434, "VISA Refnum in"=w4435) -> ()  [unwired: 10 in]
                          }
                          frame #3 {
                            n4024 = local read "VISA Refnum in\nfor Pump"() -> (w4436:refnum<visa-resource-name>)
                            n4025 = call "ProcessCompletionWaiter (SubVI).vi"("VISA Refnum in"=w4436) -> ()  [unwired: 11 in]
                          }
                          frame #4 {
                            # "External vale is temporarily connected to teh waste outlet in this code"
                            n4026 = local write "Valve V3 Open"(FALSE ("Valve V3 Open")) -> ()
                            n4027 = local write "Valve V4 Open"(FALSE ("Valve V4 Open")) -> ()
                            n4028 = local write "Valve V1 Open"(FALSE ("Valve V1 Open")) -> ()
                            n4029 = local write "Valve V2 Open"(FALSE ("Valve V2 Open")) -> ()
                            n4030 = local write "External Valve \nOpen"(FALSE ("External Valve \nOpen")) -> ()
                            n4031 = local write "Valve V8 Open"(TRUE ("Valve V8 Open")) -> ()
                            n4032 = local write "Valve V6 Open"(FALSE ("Valve V6 Open")) -> ()
                            n4033 = local write "Valve V5 Open"(FALSE ("Valve V5 Open")) -> ()
                            n4034 = local write "Valve V7 Open"(FALSE ("Valve V7 Open")) -> ()
                          }
                          frame #5 {
                            n4035 = local read "Apparent Volume\nof Syringe"() -> (w4446:dbl)
                            n4036 = local read "Buffer-B Volume \nfor elution tubing \npre-wash"() -> (w4449:dbl)
                            n4037 = Quotient & Remainder(x=w4449, y=w4446) -> (x-y*floor(x/y)=w4447:dbl, floor(x/y)=w4448:dbl)
                            n4038 = for {
                              N: w4448 -> [_]
                              n4039 = stacked-sequence {
                                frame #0 {
                                n4040 = local read "Buffer-B PickUp \nFlow Rate (ul/min)"() -> (w4452:dbl)
                                n4041 = local read "Buffer-B Pumping\nResolution"() -> (w4451:T2)
                                n4042 = local read "VISA Refnum in\nfor Pump"() -> (w4454:refnum<visa-resource-name>)
                                n4043 = local read "Apparent Volume\nof Syringe"() -> (w4450:dbl)
                                n4044 = local read "Volume of Syringe"() -> (w4453:dbl)
                                n4045 = call "RPickUp(SubVI).vi"("Volume to be picked up"=w4450, "Volume of Syringe"=w4453, "Resolution of PickUP"=w4451, "PickUp Flow Rate (ul/min)"=w4452, "VISA Refnum in"=w4454) -> ()  [unwired: 6 in, 1 out]
                                }
                                frame #1 {
                                n4046 = while {
                                stop <- w4455 stop-if-true
                                n4047 = local read "Stopper that ends \nthe main loops"() -> (w4456:bool)
                                n4048 = local read "VISA Refnum in\nfor Pump"() -> (w4457:refnum<visa-resource-name>)
                                n4049 = case shown="True" w4456 {
                                frame False {
                                }
                                frame True {
                                n4050 = local read "VISA Refnum in\nfor Pump"() -> (w4458:refnum<visa-resource-name>)
                                n4051 = call "HardStopCurrentProcess (SubVI).vi"("VISA Refnum in"=w4458) -> ()  [unwired: 11 in]
                                }
                                }
                                n4052 = call "ProcessCompletionWaiterWithOutPut (SubVI).vi"("VISA Refnum in"=w4457) -> ("Boolean"=w4455:bool)  [unwired: 10 in]
                                }
                                }
                                frame #2 {
                                # "Reads the initial Plunger Position for computing the volume dispensed"
                                n4053 = local read "VISA Refnum in\nfor Pump"() -> (w4460:refnum<visa-resource-name>)
                                n4054 = call "AbsolutePlungerPosition (SubVI).vi"("VISA Refnum in"=w4460) -> ("Plunger Position"=w4459:i32)  [unwired: 10 in]
                                n4055 = local write "Initial Plunger Position"(w4459) -> ()
                                }
                                frame #3 {
                                # "Switch to Port-8"
                                # "Port-8 of the pump is conncted to elution tubing for column-1 of chip"
                                n4056 = local read "VISA Refnum in\nfor Pump"() -> (w4462:refnum<visa-resource-name>)
                                n4057 = call "PortChanger (SubVI).vi"("Port Number"="8", "VISA Refnum in"=w4462) -> ()  [unwired: 10 in]
                                }
                                frame #4 {
                                n4058 = while {
                                stop <- w4463 stop-if-true
                                n4059 = local read "Stopper that ends \nthe main loops"() -> (w4464:bool)
                                n4060 = local read "VISA Refnum in\nfor Pump"() -> (w4465:refnum<visa-resource-name>)
                                n4061 = case shown="True" w4464 {
                                frame False {
                                }
                                frame True {
                                n4062 = local read "VISA Refnum in\nfor Pump"() -> (w4466:refnum<visa-resource-name>)
                                n4063 = call "HardStopCurrentProcess (SubVI).vi"("VISA Refnum in"=w4466) -> ()  [unwired: 11 in]
                                }
                                }
                                n4064 = call "ProcessCompletionWaiterWithOutPut (SubVI).vi"("VISA Refnum in"=w4465) -> ("Boolean"=w4463:bool)  [unwired: 10 in]
                                }
                                }
                                frame #5 {
                                n4065 = local read "Buffer-B Dispense\nFlow Rate for Elution \ntubing pre-wash"() -> (w4470:dbl)
                                n4066 = local read "Buffer-B Pumping\nResolution"() -> (w4469:T2)
                                n4067 = local read "VISA Refnum in\nfor Pump"() -> (w4472:refnum<visa-resource-name>)
                                n4068 = local write "Pause Data Collection"(TRUE ("Pause Data Collection")) -> ()
                                n4069 = local read "Volume of Syringe"() -> (w4471:dbl)
                                n4070 = call "GoToAbsolutePosition(SubVI).vi"("Absolute Volume Position in Syringe (in ul)"=0.0, "Volume of Syringe"=w4471, "Resolution of Pumping"=w4469, "Flow Rate (ul/min)"=w4470, "VISA Refnum in"=w4472) -> ()  [unwired: 6 in, 1 out]
                                }
                                frame #6 {
                                n4071 = local read "VISA Refnum in\nfor Pump"() -> (w4476:refnum<visa-resource-name>)
                                n4072 = local read "Initial Plunger Position"() -> (w4475:dbl)
                                n4073 = local read "Volume of Syringe"() -> (w4473:dbl)
                                n4074 = local read "Buffer-B Pumping\nResolution"() -> (w4474:T2)
                                n4075 = while {
                                tunnel: w4475 -> [w4483]
                                tunnel: w4476 -> [w4482]
                                tunnel: w4474 -> [w4481]
                                tunnel: w4473 -> [w4480]
                                stop <- w4478 stop-if-true
                                n4076 = stacked-sequence {
                                tunnel: w4483 -> [w4490 _]
                                tunnel: w4482 -> [w4489 w4510]
                                tunnel: w4481 -> [w4488 _]
                                tunnel: w4480 -> [w4487 _]
                                tunnel: [_ w4508] -> w4478
                                frame #0 {
                                n4077 = call "AbsolutePlungerPosition (SubVI).vi"("VISA Refnum in"=w4489) -> ("Plunger Position"=w4486:i32)  [unwired: 10 in]
                                n4078 = case shown="\"Standard Pumping\", Default" w4488 {
                                tunnel: w4490 -> [w4495 w4504]
                                tunnel: w4486 -> [w4496 w4503]
                                tunnel: [w4494 w4501] -> w4485
                                tunnel: w4487 -> [w4493 w4502]
                                frame "Standard Pumping", Default {
                                n4079 = Subtract(x=w4495, y=w4496) -> (x-y=w4492:dbl)
                                n4080 = Absolute Value(x=w4492) -> (abs(x)=w4491:dbl)
                                n4081 = Multiply(x=w4491, y=w4493) -> (x*y=w4498:dbl)
                                n4082 = Divide(x=w4498, y=3000.0) -> (x/y=w4494:dbl)
                                }
                                frame "High Resolution Pumping" {
                                n4083 = Subtract(x=w4504, y=w4503) -> (x-y=w4500:dbl)
                                n4084 = Absolute Value(x=w4500) -> (abs(x)=w4499:dbl)
                                n4085 = Multiply(x=w4499, y=w4502) -> (x*y=w4506:dbl)
                                n4086 = Divide(x=w4506, y=24000.0) -> (x/y=w4501:dbl)
                                }
                                }
                                n4087 = local write "Volume being Injected \nin this process"(w4485) -> ()
                                }
                                frame #1 {
                                n4088 = call "LSPOneStatus (SubVI).vi"("VISA Refnum in"=w4510) -> ("read buffer"=w4512:string)  [unwired: 10 in]
                                n4089 = call <vilib>:"Trim Whitespace.vi"("string"=w4512) -> ("trimmed string"=w4511:string)  [unwired: 1 in]
                                n4090 = local read "Stopper that ends \nthe main loops"() -> (w4507:bool)
                                n4091 = Equal?(x=w4511, y="/0`\u0003") -> (x = y?=w4509:bool)
                                n4092 = Or(x=w4509, y=w4507) -> (x .or. y?=w4508:bool)
                                }
                                }
                                n4093 = Wait (ms)(milliseconds to wait=u32 100) -> ()  [unwired: 1 out]
                                n4094 = local read "Stopper that ends \nthe main loops"() -> (w4477:bool)
                                n4095 = case shown="True" w4477 {
                                frame False {
                                }
                                frame True {
                                n4096 = local read "VISA Refnum in\nfor Pump"() -> (w4484:refnum<visa-resource-name>)
                                n4097 = call "HardStopCurrentProcess (SubVI).vi"("VISA Refnum in"=w4484) -> ()  [unwired: 11 in]
                                }
                                }
                                }
                                }
                                frame #7 {
                                # "Change the pump port back to Buffer-B"
                                n4098 = local read "VISA Refnum in\nfor Pump"() -> (w4515:refnum<visa-resource-name>)
                                n4099 = local read "Port for \nB-Elution"() -> (w4514:string)
                                n4100 = local write "Pause Data Collection"(TRUE ("Pause Data Collection")) -> ()
                                n4101 = Wait (ms)(milliseconds to wait=u32 500) -> ()  [unwired: 1 out]
                                n4102 = call "PortChanger (SubVI).vi"("Port Number"=w4514, "VISA Refnum in"=w4515) -> ()  [unwired: 10 in]
                                }
                                frame #8 {
                                n4103 = local read "VISA Refnum in\nfor Pump"() -> (w4518:refnum<visa-resource-name>)
                                n4104 = local write "Volume being Injected \nin this process"(0.0 ("Volume being Injected \nin this process")) -> ()
                                n4105 = call "ProcessCompletionWaiter (SubVI).vi"("VISA Refnum in"=w4518) -> ()  [unwired: 11 in]
                                }
                              }
                            }
                            n4106 = local write "Reminder of the \nVolume to be \nPumped"(w4447) -> ()
                          }
                          frame #6 {
                            n4107 = stacked-sequence {
                              frame #0 {
                                n4108 = local read "Buffer-B PickUp \nFlow Rate (ul/min)"() -> (w4522:dbl)
                                n4109 = local read "Buffer-B Pumping\nResolution"() -> (w4521:T2)
                                n4110 = local read "VISA Refnum in\nfor Pump"() -> (w4524:refnum<visa-resource-name>)
                                n4111 = local read "Reminder of the \nVolume to be \nPumped"() -> (w4520:dbl)
                                n4112 = local read "Volume of Syringe"() -> (w4523:dbl)
                                n4113 = call "RPickUp(SubVI).vi"("Volume to be picked up"=w4520, "Volume of Syringe"=w4523, "Resolution of PickUP"=w4521, "PickUp Flow Rate (ul/min)"=w4522, "VISA Refnum in"=w4524) -> ()  [unwired: 6 in, 1 out]
                              }
                              frame #1 {
                                n4114 = while {
                                stop <- w4525 stop-if-true
                                n4115 = local read "Stopper that ends \nthe main loops"() -> (w4526:bool)
                                n4116 = local read "VISA Refnum in\nfor Pump"() -> (w4527:refnum<visa-resource-name>)
                                n4117 = case shown="True" w4526 {
                                frame False {
                                }
                                frame True {
                                n4118 = local read "VISA Refnum in\nfor Pump"() -> (w4528:refnum<visa-resource-name>)
                                n4119 = call "HardStopCurrentProcess (SubVI).vi"("VISA Refnum in"=w4528) -> ()  [unwired: 11 in]
                                }
                                }
                                n4120 = call "ProcessCompletionWaiterWithOutPut (SubVI).vi"("VISA Refnum in"=w4527) -> ("Boolean"=w4525:bool)  [unwired: 10 in]
                                }
                              }
                              frame #2 {
                                # "Reads the initial Plunger Position for computing the volume dispensed"
                                n4121 = local read "VISA Refnum in\nfor Pump"() -> (w4530:refnum<visa-resource-name>)
                                n4122 = call "AbsolutePlungerPosition (SubVI).vi"("VISA Refnum in"=w4530) -> ("Plunger Position"=w4529:i32)  [unwired: 10 in]
                                n4123 = local write "Initial Plunger Position"(w4529) -> ()
                              }
                              frame #3 {
                                # "Switch to Port-8"
                                # "Port-8 of the pump is conncted to elution inlet of column-1 of chip"
                                n4124 = local read "VISA Refnum in\nfor Pump"() -> (w4532:refnum<visa-resource-name>)
                                n4125 = call "PortChanger (SubVI).vi"("Port Number"="8", "VISA Refnum in"=w4532) -> ()  [unwired: 10 in]
                              }
                              frame #4 {
                                n4126 = while {
                                stop <- w4533 stop-if-true
                                n4127 = local read "Stopper that ends \nthe main loops"() -> (w4534:bool)
                                n4128 = local read "VISA Refnum in\nfor Pump"() -> (w4535:refnum<visa-resource-name>)
                                n4129 = case shown="True" w4534 {
                                frame False {
                                }
                                frame True {
                                n4130 = local read "VISA Refnum in\nfor Pump"() -> (w4536:refnum<visa-resource-name>)
                                n4131 = call "HardStopCurrentProcess (SubVI).vi"("VISA Refnum in"=w4536) -> ()  [unwired: 11 in]
                                }
                                }
                                n4132 = call "ProcessCompletionWaiterWithOutPut (SubVI).vi"("VISA Refnum in"=w4535) -> ("Boolean"=w4533:bool)  [unwired: 10 in]
                                }
                              }
                              frame #5 {
                                n4133 = local read "Buffer-B Dispense\nFlow Rate for Elution \ntubing pre-wash"() -> (w4540:dbl)
                                n4134 = local read "Buffer-B Pumping\nResolution"() -> (w4539:T2)
                                n4135 = local read "VISA Refnum in\nfor Pump"() -> (w4542:refnum<visa-resource-name>)
                                n4136 = local write "Pause Data Collection"(TRUE ("Pause Data Collection")) -> ()
                                n4137 = local read "Volume of Syringe"() -> (w4541:dbl)
                                n4138 = call "GoToAbsolutePosition(SubVI).vi"("Absolute Volume Position in Syringe (in ul)"=0.0 ("Volume to be Dispensed"), "Volume of Syringe"=w4541, "Resolution of Pumping"=w4539, "Flow Rate (ul/min)"=w4540, "VISA Refnum in"=w4542) -> ()  [unwired: 6 in, 1 out]
                              }
                              frame #6 {
                                n4139 = local read "VISA Refnum in\nfor Pump"() -> (w4546:refnum<visa-resource-name>)
                                n4140 = local read "Initial Plunger Position"() -> (w4545:dbl)
                                n4141 = local read "Volume of Syringe"() -> (w4543:dbl)
                                n4142 = local read "Buffer-B Pumping\nResolution"() -> (w4544:T2)
                                n4143 = while {
                                tunnel: w4545 -> [w4553]
                                tunnel: w4546 -> [w4552]
                                tunnel: w4544 -> [w4551]
                                tunnel: w4543 -> [w4550]
                                stop <- w4548 stop-if-true
                                n4144 = stacked-sequence {
                                tunnel: w4553 -> [w4560 _]
                                tunnel: w4552 -> [w4559 w4580]
                                tunnel: w4551 -> [w4558 _]
                                tunnel: w4550 -> [w4557 _]
                                tunnel: [_ w4578] -> w4548
                                frame #0 {
                                n4145 = call "AbsolutePlungerPosition (SubVI).vi"("VISA Refnum in"=w4559) -> ("Plunger Position"=w4556:i32)  [unwired: 10 in]
                                n4146 = case shown="\"Standard Pumping\", Default" w4558 {
                                tunnel: w4560 -> [w4565 w4574]
                                tunnel: w4556 -> [w4566 w4573]
